vi "EmptyCSV.vi"(9 "all rows":dbl[][](array[numeric]), 10 "element":dbl, 11 "base path":path) -> (0 "error out":errorcluster)   [LabVIEW 2017]
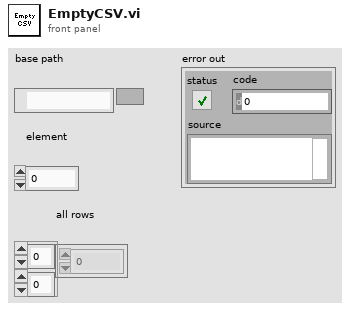
[diagram p1: front panel]
types:
  T1 = enum16{"open", "replace", "create", "open or create", "replace or create", "replace or create with confirmation"}
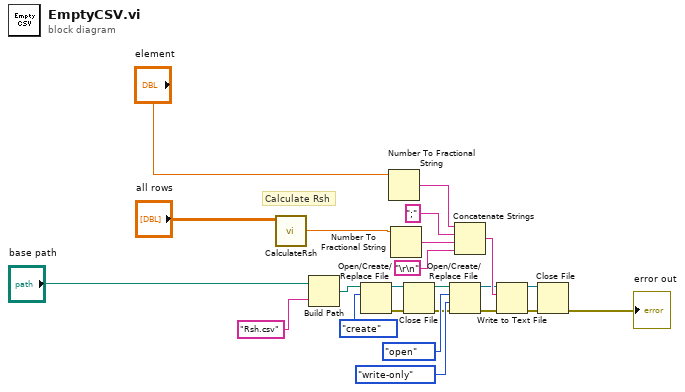
[diagram p0: block diagram]
diagram:
  # "Calculate Rsh"
  n1 = call "CalculateRsh.vi"("Array"="all rows") -> ("Rsh (Ohm)"=w21:dbl)  [unwired: 10 in]
  n2 = Build Path(base path="base path", name or relative path="Rsh.csv") -> (appended path=w2:path)
  n3 = Open/Create/Replace File(file path (use dialog)=w2, operation (0:open)=T1."create") -> (refnum out=w5:refnum<file>, error out=w4:errorcluster)  [unwired: 4 in, 1 out]
  n4 = Number To Fractional String(number="element") -> (F-format string=w22:string)  [unwired: 3 in]
  n5 = Number To Fractional String(number=w21) -> (F-format string=w18:string)  [unwired: 3 in]
  n6 = Close File(refnum=w5, error in=w4) -> (path=w11:path, error out=w12:errorcluster)
  n7 = Open/Create/Replace File(file path (use dialog)=w11, error in=w12, operation (0:open)=T1."open", access (0:read/write)=enum16{"read/write", "read-only", "write-only"}."write-only") -> (refnum out=w7:refnum<file>, error out=w8:errorcluster)  [unwired: 2 in, 1 out]
  n8 = Concatenate Strings(w22, ";" ("string"), w18, "\r\n") -> (w20:string)
  n9 = Write to Text File(file (use dialog)=w7, text=w20, error in=w8) -> (refnum out=w9:refnum<file>, error out=w10:errorcluster)  [unwired: 1 in, 1 out]
  n10 = Close File(refnum=w9, error in=w10) -> (error out=→"error out":errorcluster)  [unwired: 1 out]
